vi "test.vi"() -> ()   [LabVIEW 2012]
uses:
  clearvolume/clearvolume.lvlib
panel:
  in  "Pick your favourite backend":u32(ring) items=["USEBEST", "CUDA", "OPENCL"]
  in  "stop":bool
  out "Full Path to VI or executable":path
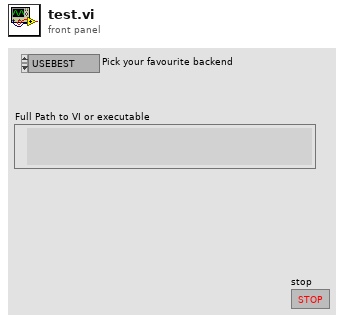
[diagram p1: front panel]
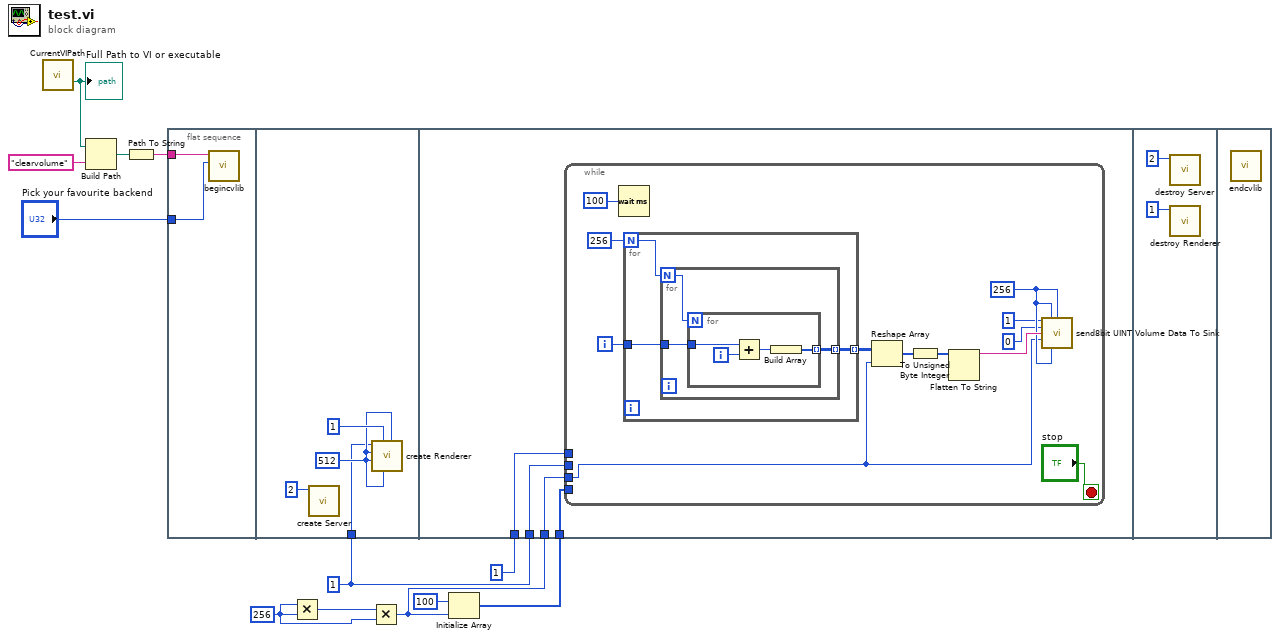
[diagram p0: block diagram]
diagram:
  w8 = i64 256 ("dimension size")
  w7 = 1 ("pRendererId")
  n1 = call "CurrentVIPath.vi"() -> ("VI or executable installation directory"=w3:path)  [unwired: 14 in, 1 out]
  "Full Path to VI or executable" <- w3
  n2 = Build Path(base path=w3, name or relative path="clearvolume") -> (appended path=w2:path)
  n3 = Path To String(path=w2) -> (string=w5:string)
  n4 = flat-sequence {
    tunnel: w5 -> [w14]
    tunnel: "Pick your favourite backend" -> [w13]
    tunnel: w7 -> [w16]
    tunnel: w10 -> [w22]
    tunnel: w9 -> [w21]
    tunnel: w7 -> [w20]
    tunnel: 1 ("pRendererId") -> [w19]
    frame #0 {
      n5 = call "begincvlib.vi"("backend"=w13, "ClearVolumeJarPath"=w14) -> ()  [unwired: 7 in, 3 out]
    }
    frame #1 {
      w17 = 512 ("pWindowWidth")
      n6 = call "create Server.vi"("pServerId"=2) -> ()  [unwired: 9 in, 2 out]
      n7 = call "create Renderer.vi"("pMaxTextureHeight"=w17, "pMaxTextureWidth"=w17, "pBytesPerVoxel"=1, "pWindowHeight"=w17, "pWindowWidth"=w17, "pRendererId"=w16) -> ()  [unwired: 4 in, 2 out]
    }
    frame #2 {
      n8 = while {
        tunnel: w22 -> [w23]
        tunnel: w21 -> [_]
        tunnel: w20 -> [_]
        tunnel: w19 -> [_]
        i -> [w30]
        stop <- "stop" stop-if-true
        w27 = 256 ("pRendererId")
        n9 = Wait (ms)(milliseconds to wait=u32 100) -> ()  [unwired: 1 out]
        n10 = for {
          N: 256 -> [w37]
          tunnel: [w36] -> w32 mode=indexing
          tunnel: w30 -> [w35]
          n11 = for {
            N: w37 -> [w40]
            tunnel: [w39] -> w36 mode=indexing
            tunnel: w35 -> [w38]
            n12 = for {
              N: w40 -> [_]
              tunnel: [w44] -> w39 mode=indexing
              tunnel: w38 -> [w43]
              i -> [w42]
              n13 = Add(x=w43, y=w42) -> (x+y=w41:i32)
              n14 = Build Array(w41) -> (w44:i32[])
            }
          }
        }
        n15 = Reshape Array(w32, w23) -> (w33:i32[])
        n16 = To Unsigned Byte Integer(number=w33) -> (unsigned 8bit integer=w29:u8[])
        n17 = Flatten To String(anything=w29) -> (data string=w28:string)  [unwired: 3 in, 2 out]
        n18 = call "send8bit UINT Volume Data To Sink.vi"("pSinkId"=1, "pWidthInVoxels"=w27, "pDepthInVoxels"=w27, "pChannelId"=0, "pBufferAddress"=w28, "pBufferLength"=w23, "pHeightInVoxels"=w27) -> ()  [unwired: 6 in, 3 out]
      }
    }
    frame #3 {
      n19 = call "destroy Server.vi"("pServerId"=2) -> ()  [unwired: 9 in, 2 out]
      n20 = call "destroy Renderer.vi"("pRendererId"=1) -> ()  [unwired: 9 in, 2 out]
    }
    frame #4 {
      n21 = call "endcvlib.vi"() -> ()  [unwired: 10 in, 2 out]
    }
  }
  n22 = Multiply(x=w8, y=w8) -> (x*y=w11:i64)
  n23 = Multiply(x=w11, y=w8) -> (x*y=w10:i64)
  n24 = Initialize Array(u8 100 ("pRendererId"), w10) -> (w9:u8[])
